vi "wczytajListePunktow.vi"(4 "Wymus generowanie punktow":bool, 5 "Rodzaj pomiarow":T1) -> (1 "Blad":bool, 2 "Wspolrzedne katowe":i32[][](array[numeric]))   [LabVIEW 2014]
uses:
  wczytajListePunktowVIs/RodzajPomiarow.ctl
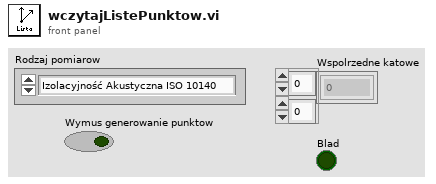
[diagram p1: front panel]
types:
  T1 = typedef "RodzajPomiarow.ctl" = enum16{"Izolacyjność Akustyczna ISO 10140", "Losowanie punktów", "Sekwencja testowa", "Definicja użytkownika"}
  T2 = typedef "WejsciaParametry.ctl" = cluster{"LEWO":bool, "PRAWO":bool, "GORA":bool, "DOL":bool, "Praca reczna":bool, "Stop":bool, "Start":bool, "Komora":bool, "Wyjscie":bool, "Rodzaj pomiarow":T1, "Czas pomiaru [s]":dbl, "Czas inicjalizacji ramion [s]":dbl, "Definicja punktów użytkownika":i32[][], "Liczba punktów":i32, "Liczba płaszczyzn":i32}
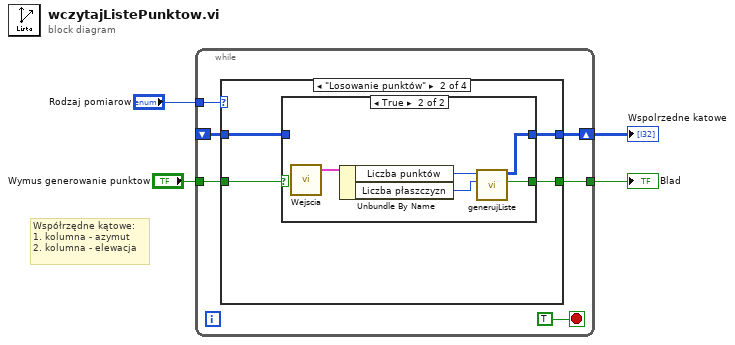
[diagram p0: block diagram]
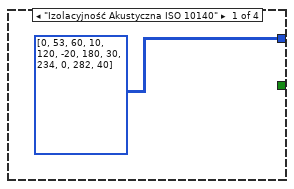
[diagram p2: hidden frame]
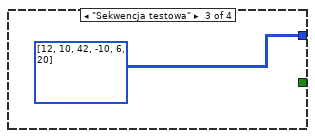
[diagram p4: hidden frame]
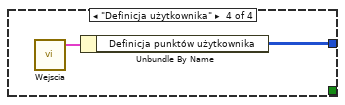
[diagram p5: hidden frame]
diagram:
  # "Współrzędne kątowe:\n1. kolumna - azymut\n2. kolumna - elewacja"
  n1 = while {
    tunnel: "Rodzaj pomiarow" -> [w9]
    shift-right: [w10] -> w4
    shift-left: _ -> [w6]
    tunnel: "Wymus generowanie punktow" -> [w5]
    tunnel: [w8] -> w2
    stop <- TRUE stop-if-true
    n2 = case shown="\"Losowanie punktów\"" w9 {
      tunnel: [i32[][] [[0, 53], [60, 10], [120, -20], [180, 30], [234, 0], [282, 40]] w15 i32[][] [[12, 10], [42, -10], [6, 20]] w24] -> w10
      tunnel: [_ w14 _ _] -> w8
      tunnel: w6 -> [_ w13 _ _]
      tunnel: w5 -> [_ w12 _ _]
      frame "Izolacyjność Akustyczna ISO 10140" {
      }
      frame "Losowanie punktów" {
        n3 = case shown="True" w12 {
          selector: w12 -> [w16 _]
          tunnel: [w17 w19] -> w15
          tunnel: [w16 w18] -> w14
          tunnel: w13 -> [w17 _]
          frame False {
          }
          frame True {
            n4 = call "Wejscia.vi"() -> ("Wyjście"=w22:T2)  [unwired: 5 in]
            n5 = Unbundle By Name(w22) -> ("Liczba punktów"=w21:i32, "Liczba płaszczyzn"=w20:i32)
            n6 = call "generujListe.vi"("Plaszczyzny"=w20, "Punkty"=w21) -> ("Blad"=w18:bool, "Lista punktow pomiarowych"=w19:i32[][])  [unwired: 8 in]
          }
        }
      }
      frame "Sekwencja testowa" {
      }
      frame "Definicja użytkownika" {
        n7 = call "Wejscia.vi"() -> ("Wyjście"=w25:T2)  [unwired: 5 in]
        n8 = Unbundle By Name(w25) -> ("Definicja punktów użytkownika"=w24:i32[][])
      }
    }
  }
  "Wspolrzedne katowe" <- w4
  "Blad" <- w2
